vi "E14_Global_Variable_1.2.vi"() -> ()   [LabVIEW 2020]
uses:
  Global 1.vi
panel:
  out "Numero pasado":i32
  out "LED2":bool
  in  "stop":bool
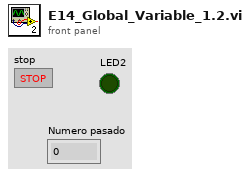
[diagram p1: front panel]
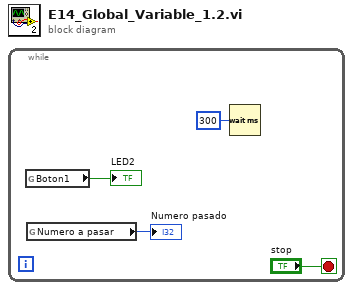
[diagram p0: block diagram]
diagram:
  n1 = while {
    stop <- "stop" stop-if-true
    n2 = global read "Global 1.vi" "Boton1"() -> (→"LED2":bool)
    n3 = global read "Global 1.vi" "Numero a pasar"() -> (→"Numero pasado":i32)
    n4 = Wait (ms)(milliseconds to wait=u32 300) -> ()  [unwired: 1 out]
  }
